vi "Launcher.vi"   [LabVIEW 2020, in "Application.lvlib" / "Application.lvclass"]
uses:
  Application.lvclass
  Application.lvclass/Application.ctl
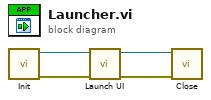
[diagram p0: block diagram]
diagram:
  n1 = call "Init.vi"() -> ("error out"=w1:errorcluster, "Application out"=w2:refnum<class "Application.lvclass">)  [unwired: 10 in]
  n2 = call "Launch UI.vi"("error in (no error)"=w1, "Application in"=w2) -> ("error out"=w3:errorcluster, "Application out"=w4:refnum<class "Application.lvclass">)  [unwired: 8 in]
  n3 = call "Close.vi"("error in (no error)"=w3, "Application in"=w4) -> ()  [unwired: 8 in, 2 out]
